vi "Read Meta Data.vi"   [LabVIEW 2015, in "NI STM.lvlib"]
doc: "This VI reads the meta data information from a remote computer. Use this VI to retrieve the variable names and types that a remote computer exports.\n\nThis VI parses the data and returns a cluster containing the meta data information.\n\nCopyright 2015, 2016, 2017 National Instruments Corporation\n\nLicensed under the Apache License, Version 2.0 (the \"License\"); you may not use this file except in compliance with the License.\n\n You may obtain a copy of the License at\n\n http://www.apache.org/licenses/LICENSE-2.0\n\nUnless required by applicable law or agreed to in writing, software distributed under the License is distributed on an \"AS IS\" BASIS, WITHOUT WARRANTIES OR CONDITIONS OF ANY KIND, either express or implied.\n\nSee the License for the specific language governing permissions and limitations under the License."
uses:
  <vilib>/NI/STM/NI STM.lvlib
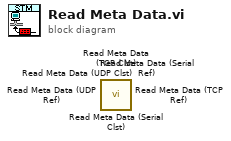
[diagram p0: block diagram]
diagram:
  n1 = call <vilib>:"Read Meta Data (Serial Clst).vi"() -> ()  [unwired: 9 in, 3 out]
  n2 = call <vilib>:"Read Meta Data (Serial Ref).vi"() -> ()  [unwired: 9 in, 3 out]
  n3 = call <vilib>:"Read Meta Data (UDP Ref).vi"() -> ()  [unwired: 8 in, 4 out]
  n4 = call <vilib>:"Read Meta Data (TCP Ref).vi"() -> ()  [unwired: 9 in, 3 out]
  n5 = call <vilib>:"Read Meta Data (UDP Clst).vi"() -> ()  [unwired: 8 in, 4 out]
  n6 = call <vilib>:"Read Meta Data (TCP Clst).vi"() -> ()  [unwired: 9 in, 3 out]
